vi "CompileCorrInfoDutNet.vi"(8 "error in (no error)":errorcluster, 11 "Device Item Ref in":T4 format="%.0x") -> (0 "error out":errorcluster, 2 "Corruption Info DUT_Network":T1 {"Frame Infos Array"."DLC Length  Corruption Index" min=-8 max=8}, 3 "Device Item Ref out":T4 format="%.0x")   [LabVIEW 2018, in "CAN Gateway System Explorer.lvlib"]
uses:
  CAN Gateway System Explorer.lvlib
  <vilib>/NI Veristand/Custom Device API/Custom Device Item Ref.ctl
  Shared/CTLs/Corruption Info.ctl
  Shared/CTLs/Frame.ctl
  Shared/CTLs/Signal_Data_Trigger.ctl
  Shared/Constants.vi
  Shared/CAN Gateway Shared.lvlib
  <vilib>/NI Veristand/Custom Device API/Custom Device API.lvlib
  Types/Frame Controls.ctl
  <vilib>/NI Veristand/Custom Device API/Get Item Property (Variant).vi
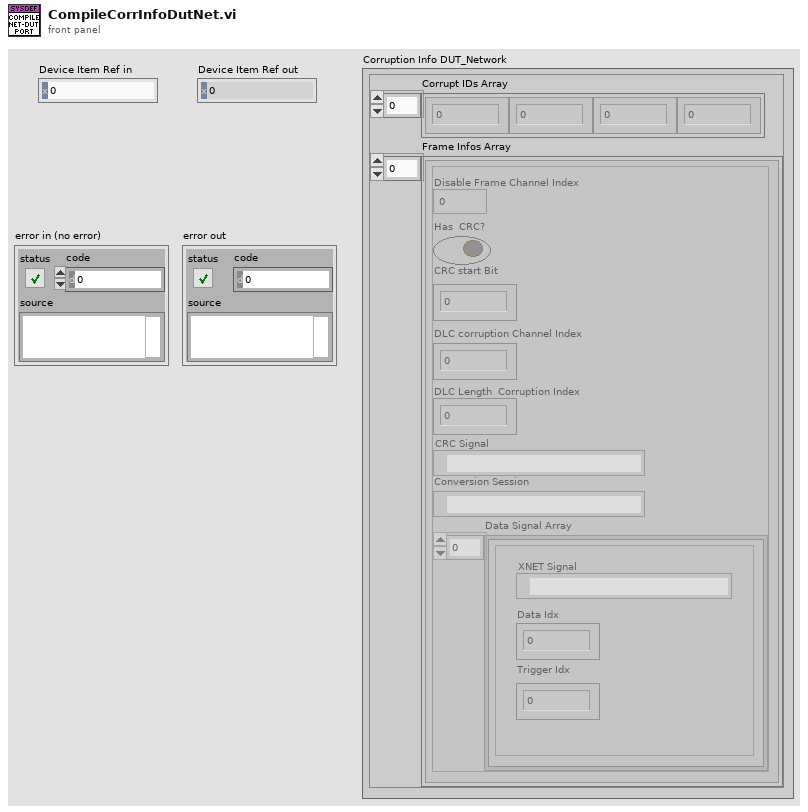
[diagram p1: front panel]
types:
  T1 = typedef "CAN Gateway Shared.lvlib/Corruption Info.ctl" = cluster{"Corrupt IDs Array":u32[], "Frame Infos Array":T2[]}
  T2 = typedef "CAN Gateway Shared.lvlib/Frame.ctl" = cluster{"Disable Frame Channel Index":i32, "Has  CRC?":bool, "CRC start Bit":u32, "DLC corruption Channel Index":i32, "DLC Length  Corruption Index":i32, "CRC Signal":refnum<k21>, "Conversion Session":refnum<k21>, "Data Signal Array":T3[]}
  T3 = typedef "CAN Gateway Shared.lvlib/Signal_Data_Trigger.ctl" = cluster{"XNET Signal":refnum<k21>, "Data Idx":u32, "Trigger Idx":u32}
  T4 = typedef "Custom Device API.lvlib/Custom Device Item Ref.ctl" = u64
  T5 = typedef "CAN Gateway System Explorer.lvlib/Frame Controls.ctl" = refnum<vi>[]
  T6 = typedef "Custom Device API.lvlib/Custom Device Item Info.ctl" = cluster{"Name":string, "Is Channel":bool, "GUID":string, "Is Waveform":bool}
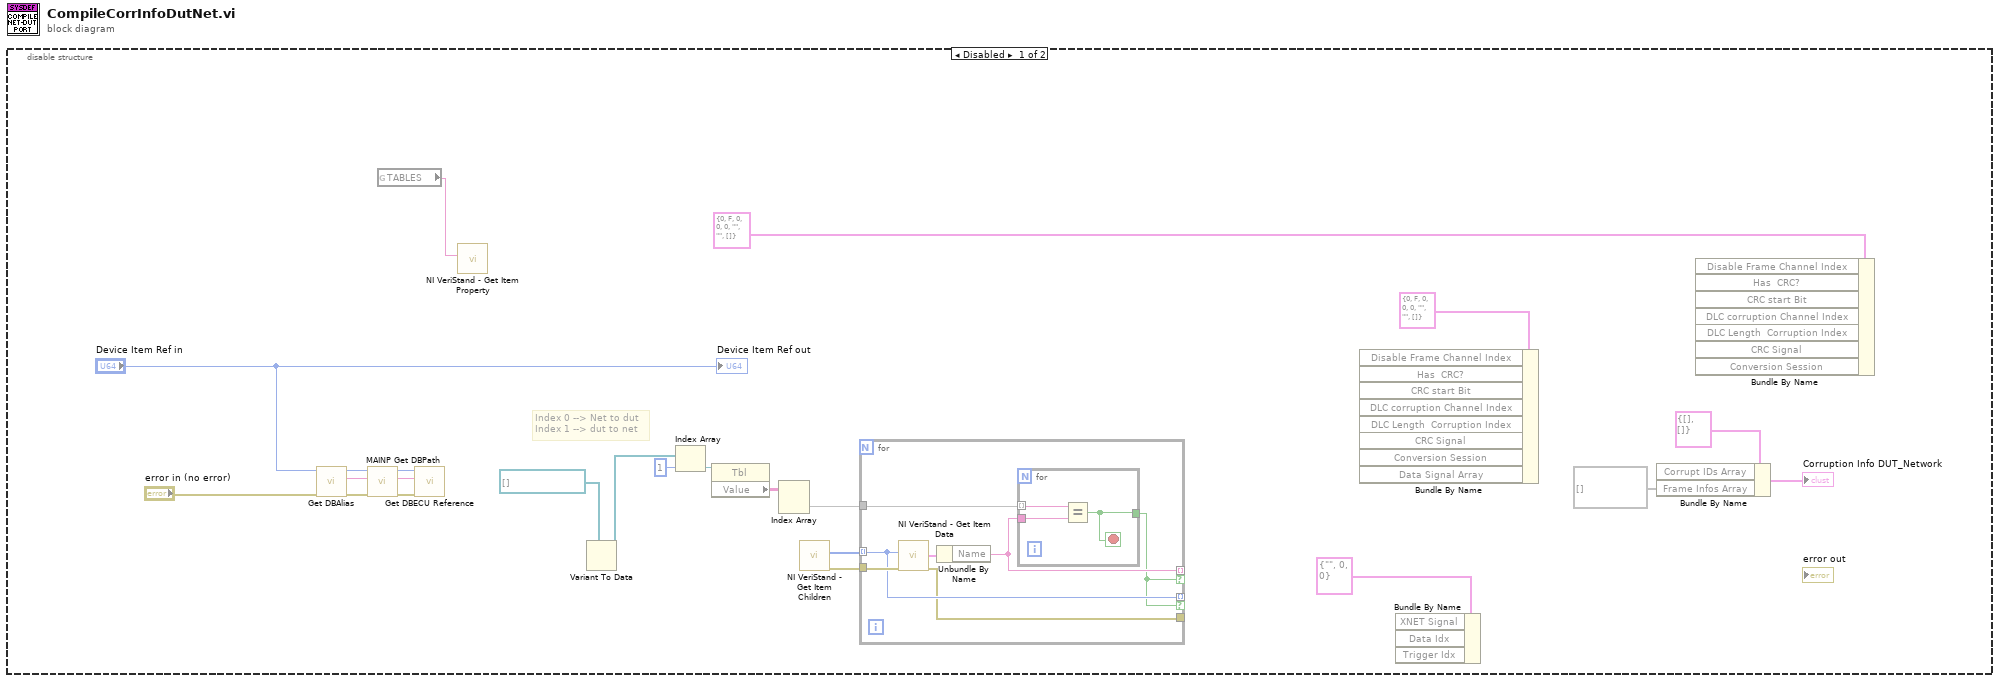
[diagram p0: block diagram]
diagram:
  n1 = disable-structure shown="Disabled" {
    frame Disabled {
      # "Index 0 --> Net to dut\nIndex 1 --> dut to net"
      n2 = call "Get DBAlias.vi"("error in (no error)"="error in (no error)", "Device Item Ref in"="Device Item Ref in") -> ("error out"=w10:errorcluster, "Alias"=w9:string, "Device Item Ref out"=w11:T4)  [unwired: 7 in]
      n3 = call "MAINP Get DBPath.vi"("error in (no error)"=w10, "Alias"=w9, "Device Item Ref in"=w11) -> ("error out"=w6:errorcluster, "Alias"=w4:string, "Device Item Ref out"=w5:T4)  [unwired: 5 in, 1 out]
      n4 = global read "Constants.vi" "TABLES"() -> (w23:string)
      n5 = call "Get DBECU Reference.vi"("error in (no error)"=w6, "Alias"=w4, "Device Item Ref in"=w5) -> ()  [unwired: 6 in, 3 out]
      n6 = call-poly <vilib>:"NI VeriStand - Get Item Property.vi"("Property Name"=w23) -> ()  [unwired: 7 in, 4 out]
      n7 = Variant To Data(type=T5 [] ("Array")) -> (data=w19:T5)  [unwired: 2 in, 1 out]
      n8 = Index Array(array=w19, index=1) -> (element=w17:refnum<vi>)
      n9 = property class="Tbl"(reference=w17) -> ("Value"=w13:string[][])  [unwired: 1 in, 2 out]
      n10 = Index Array(array=w13) -> (element=w12:string[])  [unwired: 2 in]
      n11 = call <vilib>:"NI VeriStand - Get Item Children.vi"() -> ("error out"=w14:errorcluster, "Child Refs"=w15:T4[])  [unwired: 8 in, 2 out]
      n12 = for {
        tunnel: w15 -> [w27] mode=indexing
        tunnel: w14 -> [w30]
        tunnel: w12 -> [w25]
        tunnel: [w28] -> _ mode=indexing if=w24
        tunnel: [w27] -> _ mode=indexing if=w24
        tunnel: [w26] -> _
        n13 = call <vilib>:"NI VeriStand - Get Item Data.vi"("error in (no error)"=w30, "Item Ref in"=w27) -> ("error out"=w26:errorcluster, "Item Info"=w29:T6)  [unwired: 6 in, 2 out]
        n14 = Unbundle By Name(w29) -> ("Name"=w28:string)
        n15 = for {
          tunnel: w28 -> [w33]
          tunnel: w25 -> [w32] mode=indexing
          tunnel: [w31] -> w24
          stop <- w31 stop-if-true
          n16 = Equal?(x=w32, y=w33) -> (x = y?=w31:bool)
        }
      }
      n17 = Bundle By Name(cluster=T2 {"Disable Frame Channel Index"=0, "Has  CRC?"=FALSE, "CRC start Bit"=0, "DLC corruption Channel Index"=0, "DLC Length  Corruption Index"=0, "CRC Signal"="", "Conversion Session"="", "Data Signal Array"=[]} ("Frame Infos")) -> ()  [unwired: 8 in, 1 out]
      n18 = Bundle By Name(cluster=T3 {"XNET Signal"="", "Data Idx"=0, "Trigger Idx"=0} ("Signal Data Trigger")) -> ()  [unwired: 3 in, 1 out]
      n19 = Bundle By Name(cluster=T1 {"Corrupt IDs Array"=[], "Frame Infos Array"=[]} ("Corruption Info"), "Frame Infos Array"=void[] []) -> (→"Corruption Info DUT_Network":T1)  [unwired: 1 in]
      n20 = Bundle By Name(cluster=T2 {"Disable Frame Channel Index"=0, "Has  CRC?"=FALSE, "CRC start Bit"=0, "DLC corruption Channel Index"=0, "DLC Length  Corruption Index"=0, "CRC Signal"="", "Conversion Session"="", "Data Signal Array"=[]} ("Frame Infos")) -> ()  [unwired: 7 in, 1 out]
      "Device Item Ref out" <- "Device Item Ref in"
    }
    frame Enabled {
    }
  }
